vi "axex_copy_sheet.vi"(5 "activate sheet (False)":bool, 7 "select new sheet (False)":bool, 8 "error in":errorcluster, 9 "position index (-1: last)":i32=-1, 10 "new sheet name":string, 11 "AX Excel instance in":T1) -> (0 "error out":errorcluster, 3 "AX Excel instance out":T1)   [LabVIEW 2020, in "AX Excel.lvlib"]
doc: "Call this to copy current sheet is current excel file. New sheet can be optionally selected and/or activated.\nOption 'position index' sets the position of new sheet in sheets list. Use -1 to place it to the end of list (default), 0 to place it to begining."
uses:
  AX Excel.lvlib
  axex_instance.ctl
  <vilib>/Utility/error.llb/Error Cluster From Error Code.vi
  <vilib>/ErrorRing/Error Ring.xnode
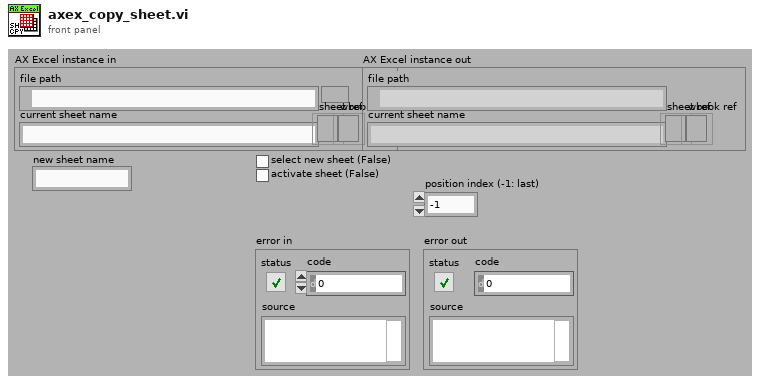
[diagram p1: front panel]
types:
  T1 = typedef "AX Excel.lvlib/axex_instance.ctl" = cluster{"file path":path, "current sheet name":string, "sheet ref":refnum<k7>, "wbook ref":refnum<k7>}
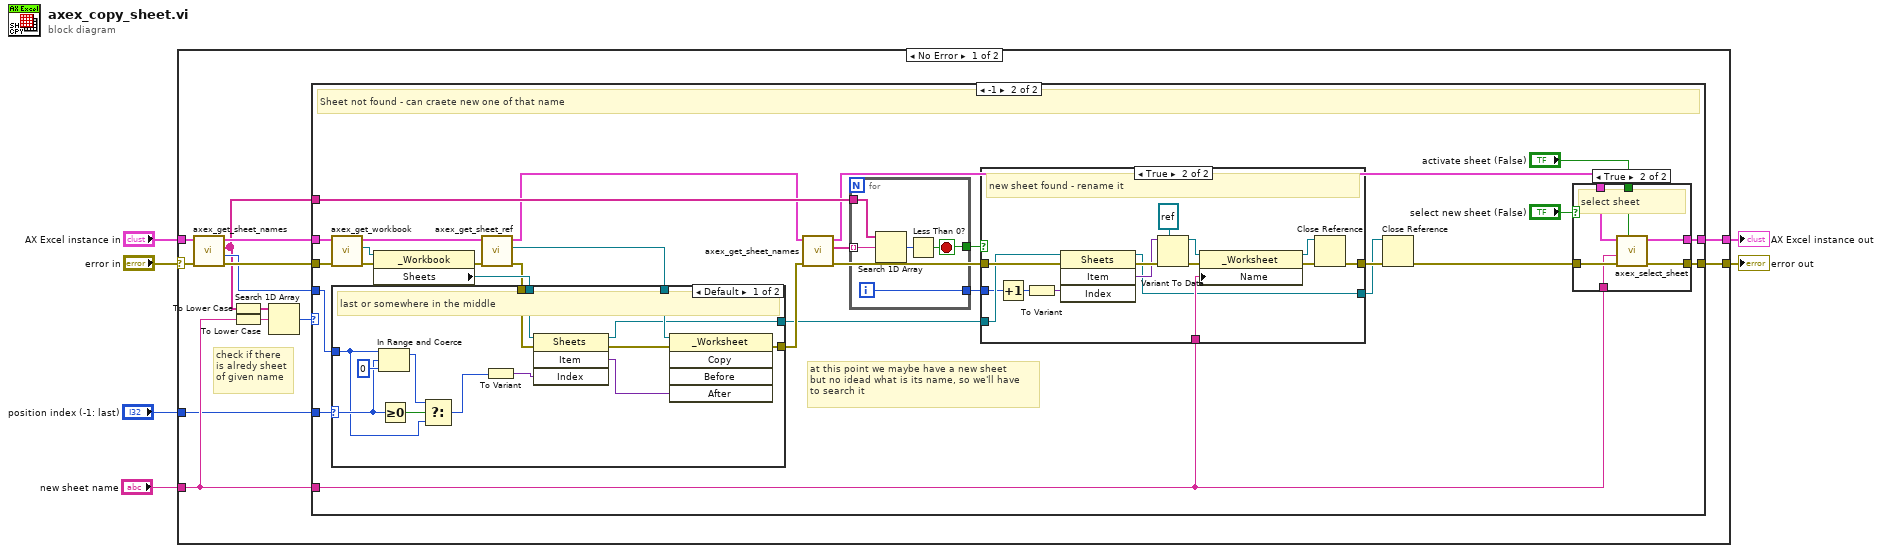
[diagram p0: block diagram]
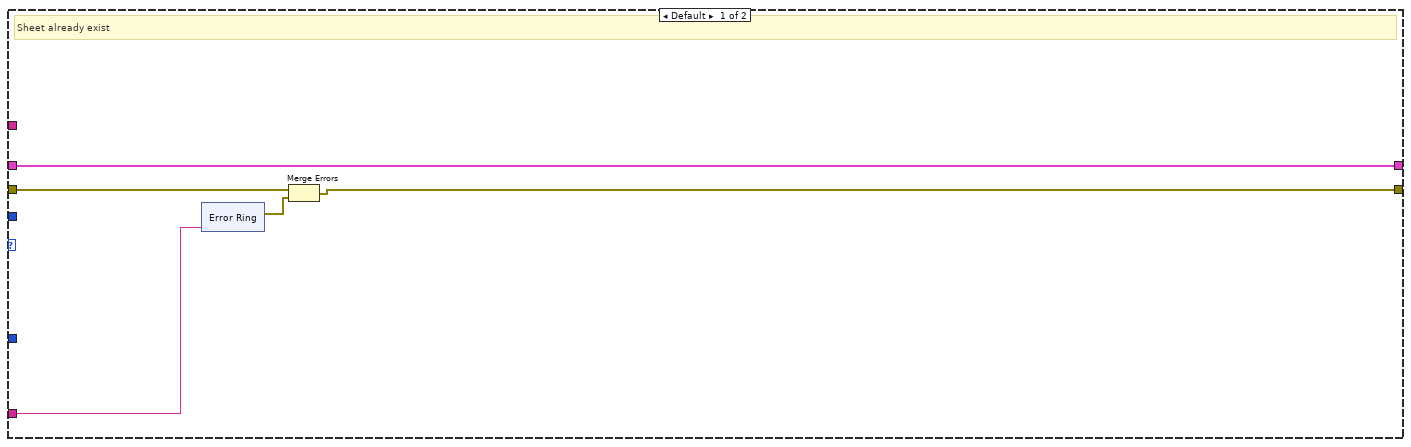
[diagram p2: hidden frame]
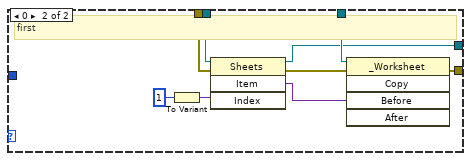
[diagram p4: hidden frame]
diagram:
  n1 = case shown="No Error" "error in" {
    selector: "error in" -> [w7 w114]
    tunnel: "AX Excel instance in" -> [w19 w113]
    tunnel: "new sheet name" -> [w13 _]
    tunnel: [w12 w113] -> w4
    tunnel: [w11 w114] -> w3
    tunnel: "position index (-1: last)" -> [w9 _]
    frame No Error {
      # "check if there\nis alredy sheet\nof given name"
      n2 = call "axex_get_sheet_names.vi"("error in"=w7, "AX Excel instance in"=w19) -> ("error out"=w15:errorcluster, "sheets count"=w10:i32, "sheet names"=w8:string[], "AX Excel instance out"=w14:T1)  [unwired: 5 in, 1 out]
      n3 = To Lower Case(string=w8) -> (all lower case string=w18:string[])
      n4 = To Lower Case(string=w13) -> (all lower case string=w17:string)
      n5 = Search 1D Array(1D array=w18, element=w17) -> (index of element=w16:i32)  [unwired: 1 in]
      n6 = case shown="-1" w16 {
        tunnel: w15 -> [w22 w59]
        tunnel: w14 -> [w24 w58]
        tunnel: w13 -> [w23 w40]
        tunnel: [w24 w55] -> w12
        tunnel: [w20 w54] -> w11
        tunnel: w10 -> [_ w50]
        tunnel: w9 -> [_ w51]
        tunnel: w8 -> [_ w47]
        frame Default {
          # "Sheet already exist"
          n7 = xnode "Error Ring"("parameter 0"=w23) -> ("error out"=w21:errorcluster)
          n8 = Merge Errors(w22, w21) -> (w20:errorcluster)
        }
        frame -1 {
          # "at this point we maybe have a new sheet\nbut no idead what is its name, so we'll have\nto search it"
          # "Sheet not found - can craete new one of that name"
          n9 = call "axex_get_workbook.vi"("error in"=w59, "AX Excel instance in"=w58) -> ("error out"=w57:errorcluster, "excel workbook"=w56:refnum<k7>, "AX Excel instance out"=w37:T1)  [unwired: 7 in]
          n10 = property class="_Workbook"(reference=w56, error in=w57) -> (error out=w39:errorcluster, "Sheets"=w49:refnum<k7>)  [unwired: 1 out]
          n11 = call "axex_get_sheet_ref.vi"("error in"=w39, "AX Excel instance in"=w37) -> ("error out"=w38:errorcluster, "sheet ref out"=w35:refnum<k7>, "AX Excel instance out"=w36:T1)  [unwired: 6 in, 1 out]
          n12 = case shown="Default" w51 {
            selector: w51 -> [w90 _]
            tunnel: w50 -> [w87 _]
            tunnel: w38 -> [w94 w98]
            tunnel: [w91 w104] -> w46
            tunnel: w49 -> [w93 w99]
            tunnel: [w83 w96] -> w42
            tunnel: w35 -> [w84 w97]
            frame Default {
              # "last or somewhere in the middle"
              n13 = In Range and Coerce(upper limit=w87, x=w90, lower limit=0) -> (coerced(x)=w88:i32)  [unwired: 1 out]
              n14 = Greater Or Equal To 0?(x=w90) -> (x >= 0?=w89:bool)
              n15 = Select(t=w88, s=w89, f=w87) -> (s? t:f=w86:i32)
              n16 = To Variant(anything=w86) -> (Variant=w85:variant)
              n17 = invoke class="Sheets" method="Item"(reference=w93, error in=w94, "Index"=w85) -> (reference out=w83:refnum<k7>, error out=w82:errorcluster, "Item"=w92:variant)  [unwired: 1 in, 1 out]
              n18 = invoke class="_Worksheet" method="Copy"(reference=w84, error in=w82, "After"=w92) -> (error out=w91:errorcluster)  [unwired: 2 in, 4 out]
            }
            frame 0 {
              # "first"
              n19 = To Variant(anything=1) -> (Variant=w101:variant)
              n20 = invoke class="Sheets" method="Item"(reference=w99, error in=w98, "Index"=w101) -> (reference out=w96:refnum<k7>, error out=w103:errorcluster, "Item"=w102:variant)  [unwired: 1 in, 1 out]
              n21 = invoke class="_Worksheet" method="Copy"(reference=w97, error in=w103, "Before"=w102) -> (error out=w104:errorcluster)  [unwired: 2 in, 4 out]
            }
          }
          n22 = call "axex_get_sheet_names.vi"("error in"=w46, "AX Excel instance in"=w36) -> ("error out"=w43:errorcluster, "sheet names"=w48:string[], "AX Excel instance out"=w45:T1)  [unwired: 5 in, 2 out]
          n23 = for {
            tunnel: w48 -> [w80] mode=indexing
            tunnel: w47 -> [w81]
            tunnel: [w78] -> w44
            tunnel: [w77] -> w41
            i -> [w77]
            stop <- w78 stop-if-true
            n24 = Search 1D Array(1D array=w81, element=w80) -> (index of element=w79:i32)  [unwired: 1 in]
            n25 = Less Than 0?(x=w79) -> (x < 0?=w78:bool)
          }
          n26 = case shown="True" w44 {
            tunnel: w43 -> [w61 w76]
            tunnel: w42 -> [w60 w75]
            tunnel: w41 -> [_ w72]
            tunnel: w40 -> [_ w64]
            tunnel: [w61 w63] -> w34
            tunnel: [w60 w62] -> w32
            frame False {
            }
            frame True {
              # "new sheet found - rename it"
              n27 = Increment(x=w72) -> (x+1=w73:i32)
              n28 = To Variant(anything=w73) -> (Variant=w74:variant)
              n29 = invoke class="Sheets" method="Item"(reference=w75, error in=w76, "Index"=w74) -> (reference out=w62:refnum<k7>, error out=w67:errorcluster, "Item"=w65:variant)  [unwired: 1 in, 1 out]
              n30 = Variant To Data(error in=w67, type=refnum<k7> refnum ("reference out"), Variant=w65) -> (data=w70:refnum<k7>, error out=w71:errorcluster)
              n31 = property class="_Worksheet"(reference=w70, error in=w71, "Name"=w64) -> (reference out=w68:refnum<k7>, error out=w69:errorcluster)
              n32 = Close Reference(reference=w68, error in (no error)=w69) -> (error out=w63:errorcluster)
            }
          }
          n33 = Close Reference(reference=w32, error in (no error)=w34) -> (error out=w33:errorcluster)
          n34 = case shown="True" "select new sheet (False)" {
            tunnel: w33 -> [w106 w112]
            tunnel: w45 -> [w105 w111]
            tunnel: [w106 w110] -> w54
            tunnel: w40 -> [_ w109]
            tunnel: [w105 w108] -> w55
            tunnel: "activate sheet (False)" -> [_ w107]
            frame False {
              # "don't select sheet"
            }
            frame True {
              # "select sheet"
              n35 = call "axex_select_sheet.vi"("activate sheet (False)"=w107, "error in"=w112, "sheet name (none)"=w109, "AX Excel instance in"=w111) -> ("error out"=w110:errorcluster, "AX Excel instance out"=w108:T1)  [unwired: 4 in, 2 out]
            }
          }
        }
      }
    }
    frame Error {
    }
  }
  "error out" <- w3
  "AX Excel instance out" <- w4
